vi "Sort Fields.vi"(10 "Message in":T1) -> (2 "Message":T1)   [LabVIEW 2024, in "LV-Protoc.lvlib" / "ProtoParser.lvclass"]
uses:
  ProtoParser.lvclass
  ProtoParser.lvclass/ProtoParser.ctl
  b177120b-8ddb-4734-a102-a70ac54d1100.vi
  LV-Proto/Proto Type.ctl
  LV-Proto/LV-Proto.lvlib
  LV-Proto/Type.ctl
  LV-Proto/Field.ctl
  LV-Proto/Message.ctl
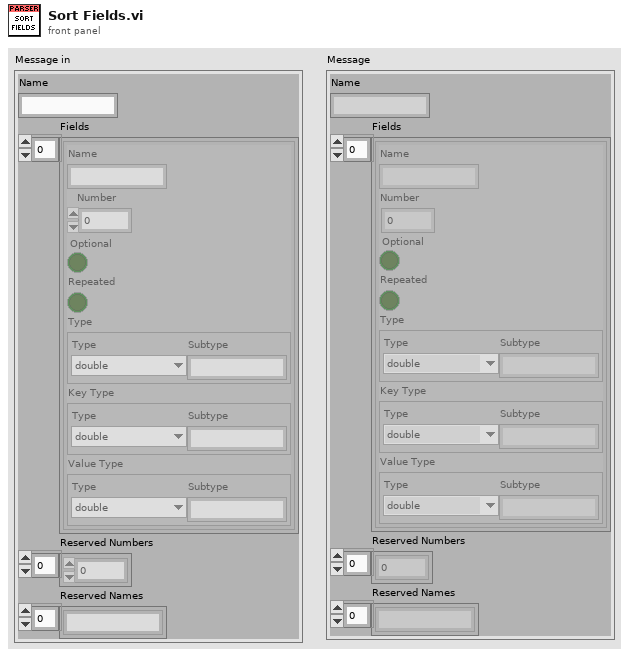
[diagram p1: front panel]
types:
  T1 = typedef "LV-Proto.lvlib/Message.ctl" = cluster{"Name":string, "Fields":T2[], "Reserved Numbers":u32[], "Reserved Names":string[]}
  T2 = typedef "LV-Proto.lvlib/Field.ctl" = cluster{"Name":string, "Number":u32, "Optional":bool, "Repeated":bool, "Type":T3, "Key Type":T3, "Value Type":T3}
  T3 = typedef "LV-Proto.lvlib/Type.ctl" = cluster{"Type":T4, "Subtype":string}
  T4 = typedef "LV-Proto.lvlib/Proto Type.ctl" = enum16{"UNKNOWN", "double", "float", "int32", "int64", "uint32", "uint64", "sint32", "sint64", "fixed32", "fixed64", "sfixed32", "sfixed64", "bool", "string", "bytes", "enum", "map", "message"}
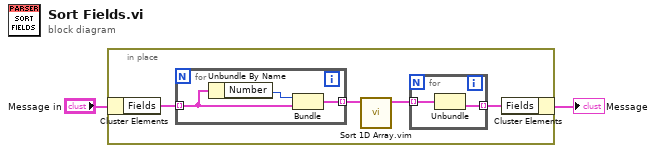
[diagram p0: block diagram]
diagram:
  n1 = in-place {
    n2 = in-place-cluster #1("Message in") -> ("Fields"=w6:T2[])
    n3 = for {
      tunnel: w6 -> [w10] mode=indexing
      tunnel: [w9] -> w5 mode=indexing
      n4 = Unbundle By Name(w10) -> ("Number"=w11:u32)
      n5 = Bundle("Number"=w11, "Field"=w10) -> (w9:cluster{"Number":u32, "Field":T2})  [unwired: 1 in]
    }
    n6 = call "Sort 1D Array.vim"("unsorted array"=w5) -> ("sorted array"=w4:cluster{"Number":u32, "Field":T2}[])  [unwired: 10 in]
    n7 = for {
      tunnel: w4 -> [w8] mode=indexing
      tunnel: [w7] -> w3 mode=indexing
      n8 = Unbundle(w8) -> ("Field"=w7:T2)  [unwired: 1 out]
    }
    n9 = in-place-cluster #1("Fields"=w3) -> (→"Message":T1)
  }
